vi "avgps.vi"(1 "data":sgl[](array[numeric])) -> (0 "Avg cts/s":dbl)   [LabVIEW 2015]
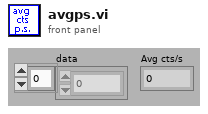
[diagram p1: front panel]
types:
  T1 = typedef "LVRectTypeDef.ctl" = cluster{"Left":i16, "Top":i16, "Right":i16, "Bottom":i16}
  T2 = cluster{"Xpixels":i32, "Vxminref":dbl, "Vxmaxref":dbl, "P":dbl, "Ypixels":i32, "Vyminref":dbl, "Vymaxref":dbl, "srate":sgl, "sAOxy":i32, "timeout":dbl, "type":string, "date":string, "time":string, "Colormap":u16, "Drawing Mode":u16, "Scanning Mode":u16, "square pixels":bool, "square matrix":bool, "Xpixels Img":i32, "Vx-min Img":dbl, "VX-max Img":dbl, "Ypixels Img":i32, "Vy-min Img":dbl, "Vy-max Img ":dbl, "Angle Img":dbl, "autoshutter":bool, "finite":bool, "cont":bool, "wavdet":bool, "measpoints":i32, "avpp":i32, "bufferAO":i32, "bufferAI":i32, "starttick":u32, "waveform":path, "Vx-ref":dbl, "Vy-ref":dbl, "refreshrate":dbl, "refreshbuffer":i32, "tt_cycles":i32, "motorref":refnum<k7>, "mirrorswitch":refnum<k7>, "sample mode":i32, "maxbufferAI":i32, "srateAODO":sgl, "bin":sgl, "Pel":sgl, "Angle draw":dbl, "srate Img":sgl, "ROIimg_plotbounds":T1, "auto OD":bool, "ODfilt":u16, "aAI":i32[], "aCI":i32[], "aAO":u32[], "aDO":u32[], "refwfsize":dbl, "Lifetime":bool, "Vz-Img":dbl, "Vz-ref":dbl, "Vz-reset":dbl, "AIoverride":bool, "aAS":u32[], "XYZstart":dbl[], "External 100KHz Clock?":bool}
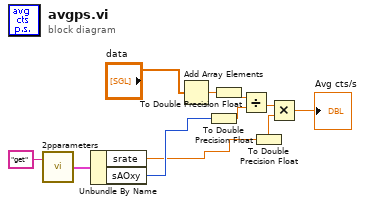
[diagram p0: block diagram]
diagram:
  n1 = call "2pparameters.vi"("command"="get") -> ("params out"=w3:T2)  [unwired: 1 in]
  n2 = Unbundle By Name(w3) -> ("srate"=w1:sgl, "sAOxy"=w2:i32)
  n3 = Add Array Elements(numeric array="data") -> (sum=w5:sgl)
  n4 = To Double Precision Float(number=w2) -> (double precision float=w8:dbl)
  n5 = To Double Precision Float(number=w5) -> (double precision float=w10:dbl)
  n6 = Divide(x=w10, y=w8) -> (x/y=w6:dbl)
  n7 = To Double Precision Float(number=w1) -> (double precision float=w9:dbl)
  n8 = Multiply(x=w6, y=w9) -> (x*y=→"Avg cts/s":dbl)
